vi "Autonomous.vi"() -> ()   [LabVIEW 2011]
uses:
  <vilib>/Instr/_visa.llb/VISA Configure Serial Port (Instr).vi
panel:
  in  "Delay (ms)":u32[](array[numeric])
  in  "Right Motor":i32[](array[numeric])
  in  "Left Motor":i32[](array[numeric])
  in  "stop":bool
  in  "baud rate (9600)":u32=115200
  in  "VISA resource name":refnum<visa-resource-name>
  out "Left Motor":i32
  out "Right Motor":i32
  in  "Autonomous Mode":bool
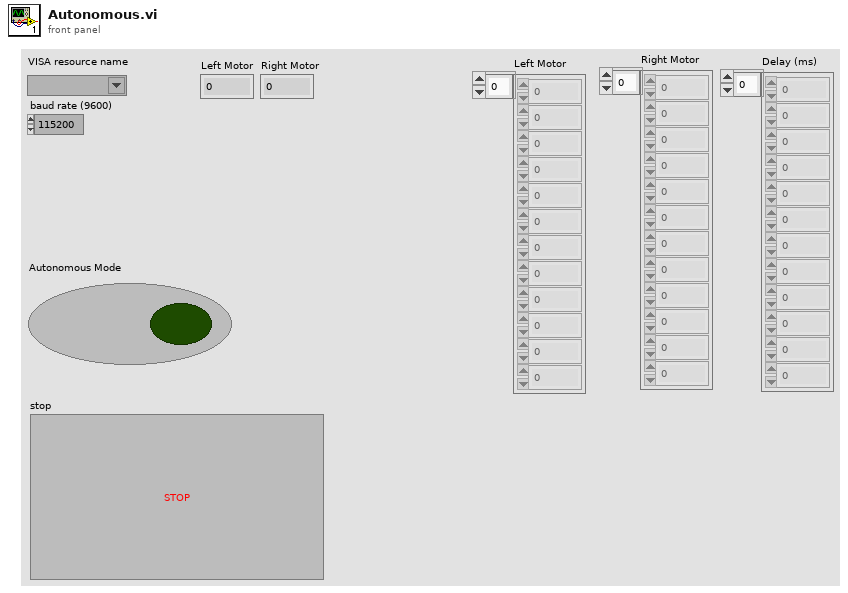
[diagram p1: front panel]
types:
  T1 = cluster{"axes total":u32, "buttons total":u32, "pov total":u32, "device name":string}[]
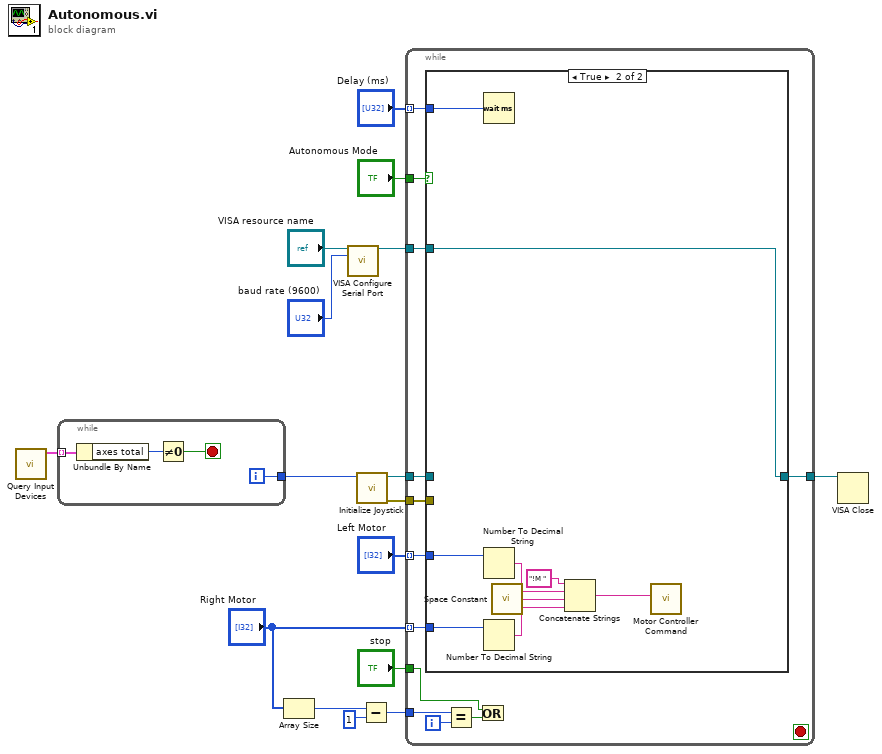
[diagram p0: block diagram]
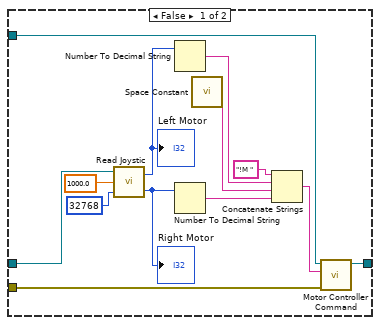
[diagram p2: hidden frame]
diagram:
  n1 = call <vilib>:"Query Input Devices.vi"() -> ("joystick info"=w16:T1)  [unwired: 8 in, 3 out]
  n2 = while {
    tunnel: w16 -> [w20] mode=indexing
    tunnel: [w17] -> w15
    i -> [w17]
    stop <- w18 stop-if-true
    n3 = Unbundle By Name(w20) -> ("axes total"=w19:u32)
    n4 = Not Equal To 0?(x=w19) -> (x != 0?=w18:bool)
  }
  n5 = Array Size(array="Right Motor") -> (size(s)=w3:i32)
  n6 = call-poly "VISA Configure Serial Port"("VISA resource name"="VISA resource name", "baud rate (9600)"="baud rate (9600)") -> ("VISA resource name out"=w11:refnum<visa-resource-name>)  [unwired: 12 in, 1 out]
  n7 = call <vilib>:"Initialize Joystick.vi"("device index"=w15) -> ("error out"=w7:errorcluster, "device ID"=w10:refnum<k1>)  [unwired: 9 in]
  n8 = Subtract(x=w3, y=1) -> (x-y=w1:i32)
  n9 = while {
    tunnel: "stop" -> [w21]
    tunnel: w11 -> [w32]
    tunnel: w10 -> [w31]
    tunnel: [w30] -> w9
    tunnel: "Autonomous Mode" -> [w29]
    tunnel: w7 -> [w28]
    tunnel: "Left Motor" -> [w27] mode=indexing
    tunnel: "Right Motor" -> [w26] mode=indexing
    tunnel: "Delay (ms)" -> [w25] mode=indexing
    tunnel: w1 -> [w24]
    i -> [w23]
    stop <- _ stop-if-true
    n10 = case shown="True" w29 {
      tunnel: w32 -> [w36 w54]
      tunnel: w31 -> [w35 _]
      tunnel: [w34 w54] -> w30
      tunnel: w28 -> [w33 _]
      tunnel: w27 -> [_ w48]
      tunnel: w26 -> [_ w47]
      tunnel: w25 -> [_ w46]
      frame False {
        n11 = call "Read Joystic.vi"("JoystickOutMaximum"=32768, "MaxMotorSpeed"=1000.0 ("HalfMaxMotorSpeed"), "device ID"=w35) -> ("Right Motor"=w41:i32, "Left Motor"=w42:i32)
        "Left Motor" <- w42
        "Right Motor" <- w41
        n12 = Number To Decimal String(number=w42) -> (decimal integer string=w40:string)  [unwired: 1 in]
        n13 = Number To Decimal String(number=w41) -> (decimal integer string=w39:string)  [unwired: 1 in]
        n14 = call <vilib>:"Space Constant.vi"() -> ("String"=w38:string)
        n15 = Concatenate Strings("!M " ("string"), w40, w38, w39) -> (w37:string)
        n16 = call "Motor Controller Command.vi"("error in (no error)"=w33, "Command"=w37, "VISA resource name"=w36) -> ("VISA resource name out"=w34:refnum<visa-resource-name>)  [unwired: 6 in, 2 out]
      }
      frame True {
        n17 = Wait (ms)(milliseconds to wait=w46) -> ()  [unwired: 1 out]
        n18 = Number To Decimal String(number=w48) -> (decimal integer string=w52:string)  [unwired: 1 in]
        n19 = Number To Decimal String(number=w47) -> (decimal integer string=w51:string)  [unwired: 1 in]
        n20 = call <vilib>:"Space Constant.vi"() -> ("String"=w50:string)
        n21 = Concatenate Strings("!M " ("string"), w52, w50, w51) -> (w49:string)
        n22 = call "Motor Controller Command.vi"("Command"=w49) -> ()  [unwired: 8 in, 3 out]
      }
    }
    n23 = Equal?(x=w24, y=w23) -> (x = y?=w22:bool)
    n24 = Or(x=w21, y=w22) -> ()  [unwired: 1 out]
  }
  n25 = VISA Close(VISA resource name=w9) -> ()  [unwired: 1 in, 1 out]
